vi "ExtendedKalmanFilter_GetP.vi"(11 "in ExtendedKalmanFiilter":T2) -> (3 "P":T1)   [LabVIEW 2019, in "Trajectory_Library.lvlib"]
doc: "Returns the error covariance matrix P.\n\nInputs:\n - inExtendedKalmanFIlter -- filter data cluster\n\nOutput: \n - P -- the error covariance matrix P."
uses:
  Trajectory_Library.lvlib
  <vilib>/Analysis/Matrix/Datatypes/RealMatrix.ctl
  <vilib>/Analysis/Matrix/NI_Matrix.lvlib
  TypeDef/EXTENDED_KALMAN_FILTER.ctl
panel:
  # "State Estimate <Statess,1>"
  # "<States, States>"
  # "<States, States>"
  # "<Statess,  States>"
  # "<Outputs, Outputs>"
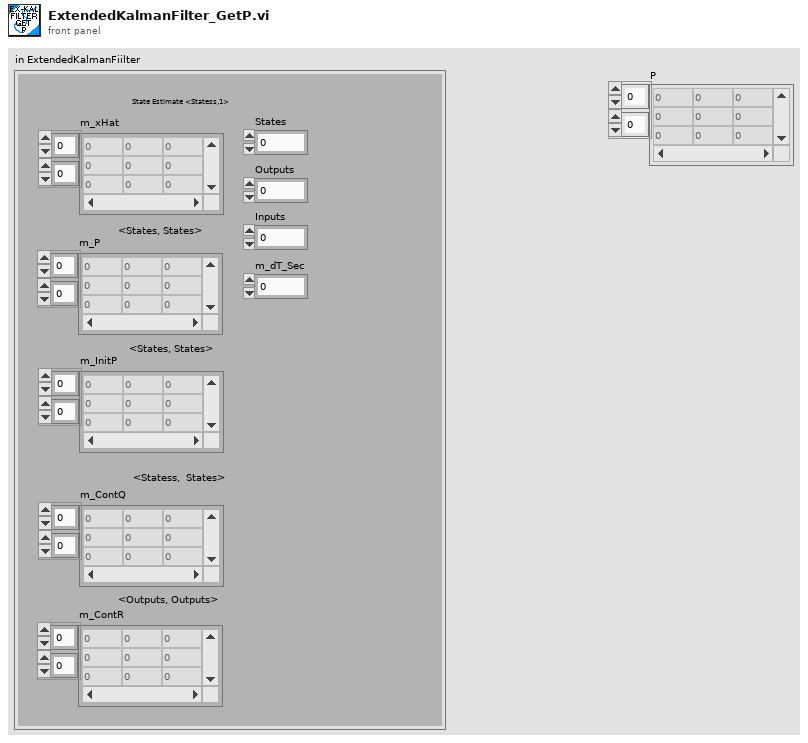
[diagram p1: front panel]
types:
  T1 = typedef "NI_Matrix.lvlib/RealMatrix.ctl" = dbl[][]
  T2 = typedef "Trajectory_Library.lvlib/EXTENDED_KALMAN_FILTER.ctl" = cluster{"m_P":T1, "m_xHat":T1, "States":i32, "Outputs":i32, "m_ContR":T1, "m_ContQ":T1, "m_dT_Sec":dbl, "Inputs":i32, "m_InitP":T1}
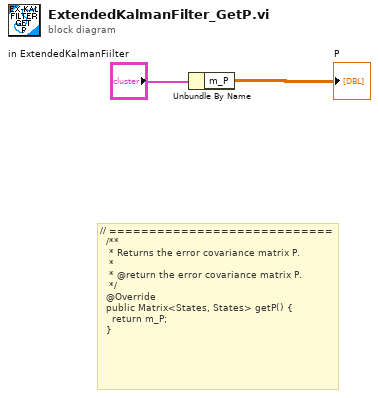
[diagram p0: block diagram]
diagram:
  # "// ============================\n  /**\n   * Returns the error covariance matrix P.\n   *\n   * @return the error covariance matrix P.\n   */\n  @Override\n  public Matrix<States, States> getP() {\n    return m_P;\n  }"
  n1 = Unbundle By Name("in ExtendedKalmanFiilter") -> ("m_P"=→"P":T1)
